vi "Handle Pumps.vi"(8 "error in (no error)":errorcluster, 11 "Stand in":refnum<class "Stand.lvclass">) -> (0 "error out":errorcluster, 3 "Stand out":refnum<class "Stand.lvclass">)   [LabVIEW 2019, in "Stand.lvclass"]
uses:
  Stand.lvclass
  Stand.lvclass/Stand.ctl
  Engine_1DI_2DO_class/Engine_1DI_2DO.lvclass
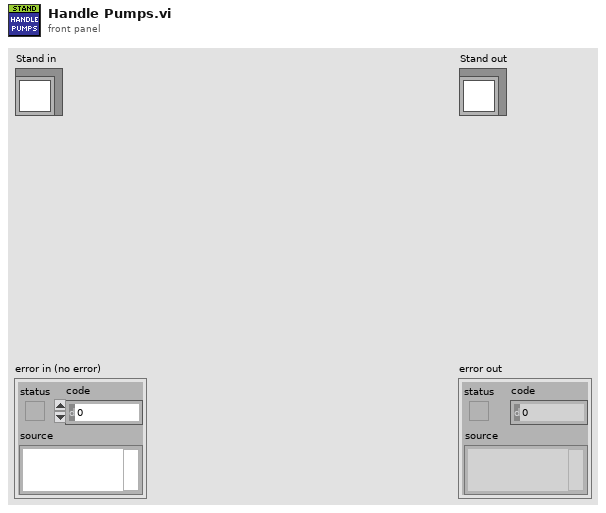
[diagram p1: front panel]
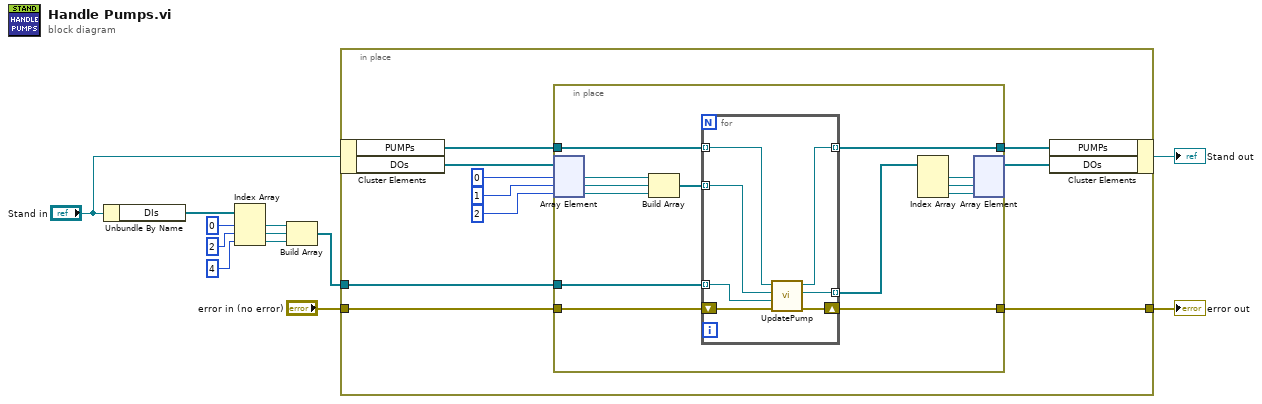
[diagram p0: block diagram]
diagram:
  n1 = Unbundle By Name("Stand in") -> ("DIs"=w10:refnum<class "Sig_DI_Simple.lvclass">[])
  n2 = Index Array(array=w10, index #1=0 ("index"), index #2=2 ("index"), index #3=4 ("index")) -> (element #1=w5:refnum<class "Sig_DI_Simple.lvclass">, element #2=w3:refnum<class "Sig_DI_Simple.lvclass">, element #3=w6:refnum<class "Sig_DI_Simple.lvclass">)
  n3 = Build Array(w5, w3, w6) -> (w4:refnum<class "Sig_DI_Simple.lvclass">[])
  n4 = in-place {
    in-place-border: w4 -> [w15]
    in-place-border: "error in (no error)" -> [w14]
    in-place-border: [w13] -> w1
    n5 = in-place-cluster #1("Stand in") -> ("PUMPs"=w22:refnum<class "Engine_1DI_2DO.lvclass">[], "DOs"=w20:refnum<class "Sig_DO_Simple.lvclass">[])
    n6 = in-place {
      in-place-border: w22 -> [w35]
      in-place-border: [w34] -> w21
      in-place-border: w15 -> [w25]
      in-place-border: w14 -> [w24]
      in-place-border: [w23] -> w13
      n7 = in-place-array #2(w20, 0, 1, 2) -> (w33:refnum<class "Sig_DO_Simple.lvclass">, w32:refnum<class "Sig_DO_Simple.lvclass">, w31:refnum<class "Sig_DO_Simple.lvclass">)
      n8 = Build Array(w33, w32, w31) -> (w30:refnum<class "Sig_DO_Simple.lvclass">[])
      n9 = for {
        tunnel: w35 -> [w42] mode=indexing
        tunnel: [w41] -> w34 mode=indexing
        tunnel: [w40] -> w29 mode=indexing
        tunnel: w30 -> [w39] mode=indexing
        tunnel: w25 -> [w38] mode=indexing
        shift-right: [w36] -> w23
        shift-left: w24 -> [w37]
        n10 = call "UpdatePump.vi"("error in (no error)"=w37, "DI"=w38, "DO in"=w39, "Pump_1AI_1DO_2DI in"=w42) -> ("error out"=w36:errorcluster, "DO out"=w40:refnum<class "Sig_DO_Simple.lvclass">, "Pump_1AI_1DO_2DI out"=w41:refnum<class "Engine_1DI_2DO.lvclass">)  [unwired: 5 in]
      }
      n11 = Index Array(array=w29) -> (element #1=w28:refnum<class "Sig_DO_Simple.lvclass">, element #2=w27:refnum<class "Sig_DO_Simple.lvclass">, element #3=w26:refnum<class "Sig_DO_Simple.lvclass">)  [unwired: 3 in]
      n12 = in-place-array #2(w28, w27, w26) -> (w19:refnum<class "Sig_DO_Simple.lvclass">[])  [unwired: 3 out]
    }
    n13 = in-place-cluster #1("PUMPs"=w21, "DOs"=w19) -> (→"Stand out":refnum<class "Stand.lvclass">)
  }
  "error out" <- w1
